vi "Arraybuilder.vi"(1 "Array in":u16[](array[numeric]), 5 "Element 1":dbl, 7 "Element 2":dbl, 9 "Element 3":dbl) -> (4 "Array out":u16[](array[numeric]))   [LabVIEW 2025]
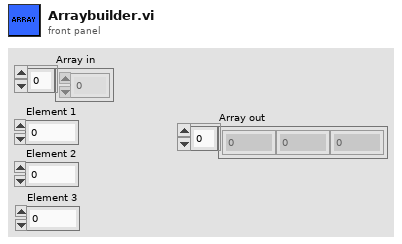
[diagram p1: front panel]
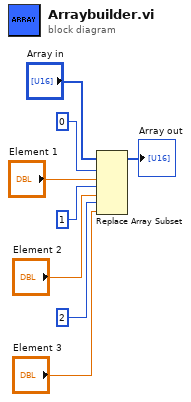
[diagram p0: block diagram]
diagram:
  n1 = Replace Array Subset(array="Array in", new element #1="Element 1", index #1=0 ("index"), new element #2="Element 2", index #2=1 ("index"), new element #3="Element 3", index #3=2 ("index")) -> (→"Array out":u16[])
